vi "Set Team Start.vi"(8 "error in (no error)":errorcluster, 9 "Set Team Start":T1, 10 "Team":refnum<class "Team.lvclass">, 11 "Game in":refnum<class "Game.lvclass">) -> (0 "error out":errorcluster, 3 "Game out":refnum<class "Game.lvclass">)   [LabVIEW 2020, in "SquareBattle.lvlib" / "Game.lvclass"]
uses:
  Game.lvclass
  Team/Team.lvclass
  Position.ctl
  Game.lvclass/Game.ctl
  SquareBattle.lvlib
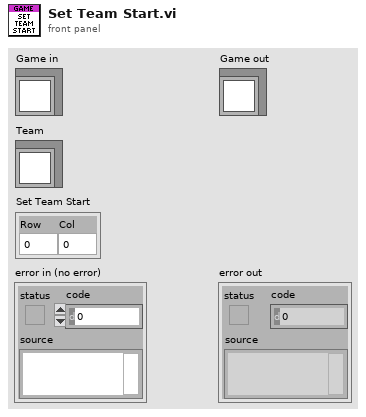
[diagram p1: front panel]
types:
  T1 = typedef "SquareBattle.lvlib/Position.ctl" = cluster{"Row":i32, "Col":i32}
  T2 = typedef "SquareBattle.lvlib/Team ID.ctl" = u32
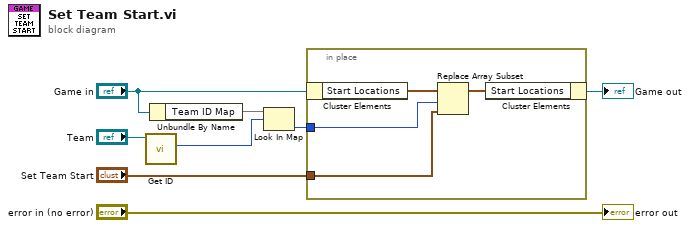
[diagram p0: block diagram]
diagram:
  n1 = call "Get ID.vi"("Team in"="Team") -> ("Team ID"=w5:T2)  [unwired: 8 in, 2 out]
  n2 = Unbundle By Name("Game in") -> ("Team ID Map"=w7:map{u32, i32})
  n3 = Look In Map(map=w7, key=w5) -> (value=w4:i32)  [unwired: 1 in, 1 out]
  n4 = in-place {
    in-place-border: w4 -> [w9]
    in-place-border: "Set Team Start" -> [w10]
    n5 = in-place-cluster #1("Game in") -> ("Start Locations"=w12:T1[])
    n6 = Replace Array Subset(array=w12, new element=w10, index=w9) -> (w11:T1[])
    n7 = in-place-cluster #1("Start Locations"=w11) -> (→"Game out":refnum<class "Game.lvclass">)
  }
  "error out" <- "error in (no error)"
